vi "CLD 14 FGV Timer.vi"(8 "Error In":errorcluster, 10 "Time Target (s) [0]":dbl, 11 "CLD 14 FGV Enum":T1) -> (0 "Error Out":errorcluster, 1 "Time Target Out":dbl, 2 "Has Time Elapsed ?":bool, 3 "Elapsed Time (s.ss)":dbl format="%#_2g", 4 "Pause ?":bool)   [LabVIEW 2009]
doc: "CLD 14 Exercise\nThis VI is used as an FGV. \nNote on reading time when in pause. The developer should not call the read time function when in pause; however, a case structure is used to defensively program the read state for this possibility."
uses:
  CLD 14 FGV Enum.ctl
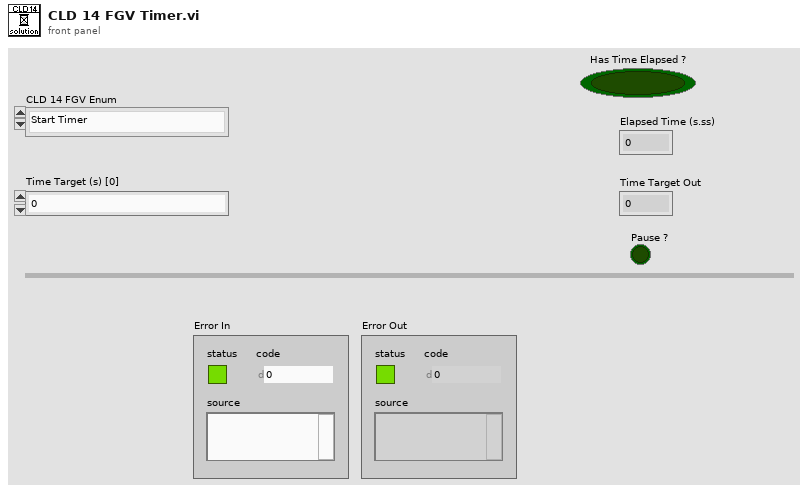
[diagram p1: front panel]
types:
  T1 = typedef "CLD 14 FGV Enum.ctl" = enum16{"Start Timer", "Read Time", "Pause", "UnPause"}
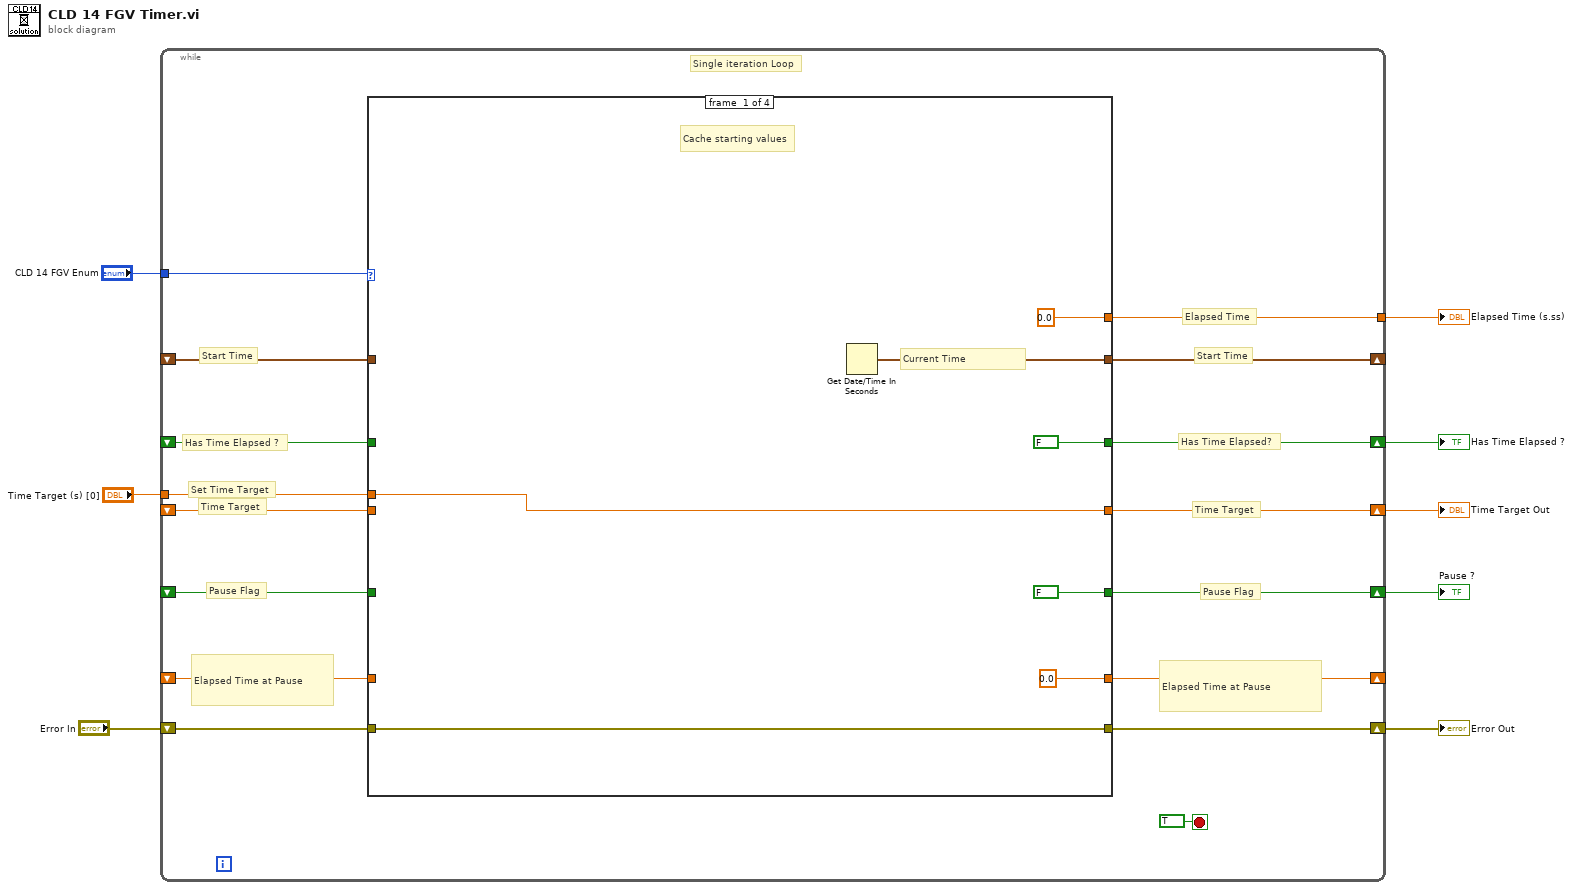
[diagram p0: block diagram]
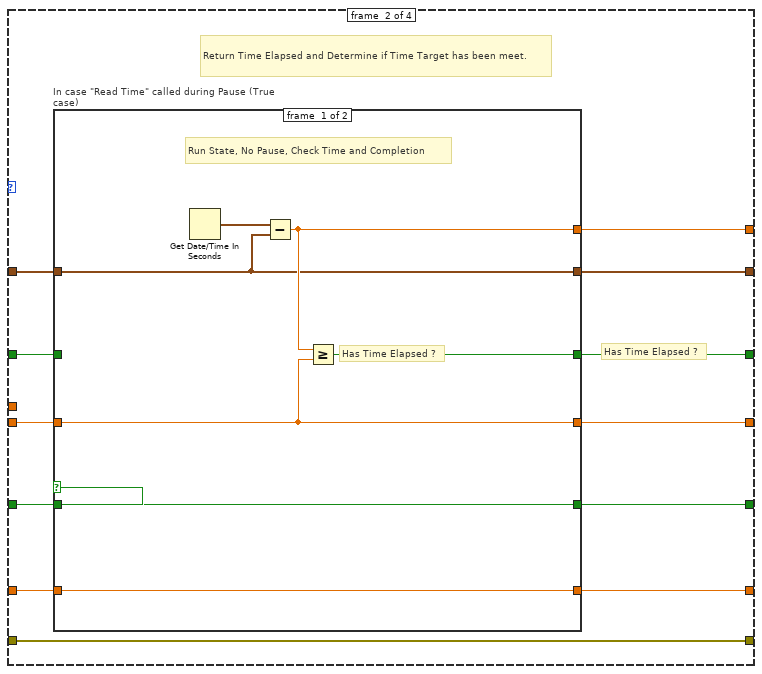
[diagram p2: hidden frame]
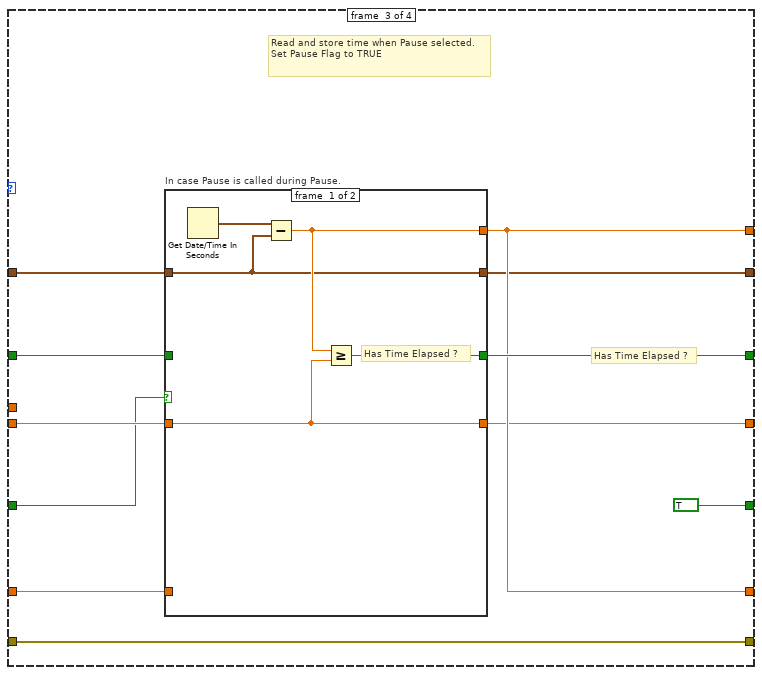
[diagram p4: hidden frame]
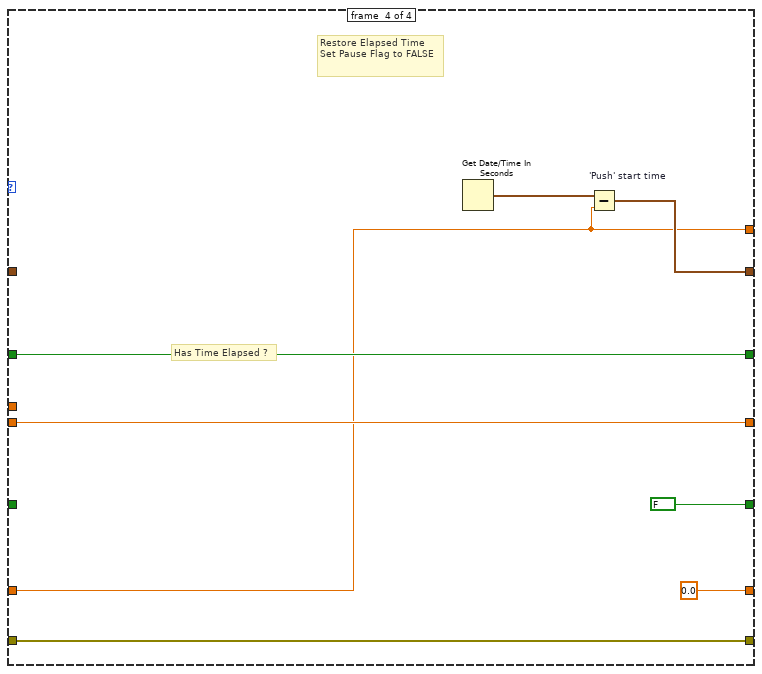
[diagram p6: hidden frame]
diagram:
  n1 = while {
    tunnel: "CLD 14 FGV Enum" -> [w24]
    shift-right: [w22] -> _
    shift-left: _ -> [w21]
    tunnel: [w20] -> w1
    shift-right: [w19] -> w7
    shift-left: "Error In" -> [w18]
    tunnel: "Time Target (s) [0]" -> [w15]
    shift-right: [w16] -> w3
    shift-left: _ -> [w17]
    shift-right: [w14] -> w4
    shift-left: _ -> [w13]
    shift-right: [w12] -> w2
    shift-left: _ -> [w11]
    shift-right: [w10] -> _
    shift-left: _ -> [w9]
    stop <- TRUE ("stop") stop-if-true
    # "Start Time"
    # "Start Time"
    # "Elapsed Time"
    # "Time Target"
    # "Time Target"
    # "Set Time Target"
    # "Has Time Elapsed?"
    # "Has Time Elapsed ?"
    # "Pause Flag"
    # "Pause Flag"
    # "Elapsed Time at Pause"
    # "Elapsed Time at Pause"
    # "Single iteration Loop"
    n2 = case shown="\"Start Timer\", Default" w24 {
      tunnel: [w31 w37 w56 w77] -> w22
      tunnel: w21 -> [_ w43 w66 _]
      tunnel: [0.0 ("Elapsed Time") w40 w61 w76] -> w20
      tunnel: [w29 w42 w65 w83] -> w19
      tunnel: w18 -> [w29 w42 w65 w83]
      tunnel: w17 -> [_ w32 w64 w82]
      tunnel: [w28 w33 w57 w82] -> w16
      tunnel: w15 -> [w28 _ _ _]
      tunnel: [FALSE w41 w63 w80] -> w14
      tunnel: w13 -> [_ w34 w60 w80]
      tunnel: [FALSE w36 TRUE FALSE] -> w12
      tunnel: w11 -> [_ w35 w59 _]
      tunnel: [0.0 w38 w61 0.0] -> w10
      tunnel: w9 -> [_ w39 w58 w76]
      frame #0 {
        # "Current Time"
        # "Cache starting values"
        n3 = Get Date/Time In Seconds() -> (seconds since 1Jan1904=w31:timestamp)
      }
      frame #1 {
        # "Has Time Elapsed ?"
        # "Return Time Elapsed and Determine if Time Target has been meet."
        n4 = case "In case \"Read Time\" called during Pause (True case)" shown="True" w35 {
          tunnel: w43 -> [w47 w55]
          tunnel: w32 -> [w46 w54]
          tunnel: [w49 w52] -> w41
          tunnel: [w48 w51] -> w40
          tunnel: w39 -> [w44 w51]
          tunnel: [w44 w51] -> w38
          tunnel: [w47 w55] -> w37
          tunnel: [w46 w54] -> w33
          tunnel: [w45 w53] -> w36
          tunnel: w35 -> [w45 w53]
          tunnel: w34 -> [_ w52]
          frame #0 {
            # "Has Time Elapsed ?"
            # "Run State, No Pause, Check Time and Completion"
            n5 = Get Date/Time In Seconds() -> (seconds since 1Jan1904=w50:timestamp)
            n6 = Subtract(x=w50, y=w47) -> (x-y=w48:dbl)
            n7 = Greater Or Equal?(x=w48, y=w46) -> (x >= y?=w49:bool)
          }
          frame #1 {
            # "Pause State, Just return Shift Registers. Do not call 'Read Time'  when in pause."
          }
        }
      }
      frame #2 {
        # "Has Time Elapsed ?"
        # "Read and store time when Pause selected.\nSet Pause Flag to TRUE"
        n8 = case "In case Pause is called during Pause." shown="True" w59 {
          tunnel: w66 -> [w67 w72]
          tunnel: w64 -> [w68 w73]
          tunnel: [w70 w75] -> w63
          tunnel: [w69 w74] -> w61
          tunnel: w60 -> [_ w75]
          tunnel: w58 -> [_ w74]
          tunnel: [w68 w73] -> w57
          tunnel: [w67 w72] -> w56
          frame #0 {
            # "Has Time Elapsed ?"
            n9 = Get Date/Time In Seconds() -> (seconds since 1Jan1904=w71:timestamp)
            n10 = Subtract(x=w71, y=w67) -> (x-y=w69:dbl)
            n11 = Greater Or Equal?(x=w69, y=w68) -> (x >= y?=w70:bool)
          }
          frame #1 {
            # "Pause called when already in pause.\n\nJust read the registers and pass out the values."
          }
        }
      }
      frame #3 {
        # "Has Time Elapsed ?"
        # "Restore Elapsed Time\nSet Pause Flag to FALSE"
        n12 = Get Date/Time In Seconds() -> (seconds since 1Jan1904=w78:timestamp)
        n13 = Subtract "'Push' start time"(x=w78, y=w76) -> (x-y=w77:timestamp)
      }
    }
  }
  "Error Out" <- w7
  "Has Time Elapsed ?" <- w4
  "Elapsed Time (s.ss)" <- w1
  "Time Target Out" <- w3
  "Pause ?" <- w2
